vi "service_template.vi"() -> ()   [LabVIEW 2010]
panel:
  in  "password":string
  in  "username":string
  out "# elements in queue":i32
  out "error out":errorcluster
  in  "attributes":string[][](array[string])
  in  "Service Name":string
  in  "Network Manager IP Address or Hostname":string
  in  "timeout ms":i32=10000
  in  "Network Manager port":u16=1875
  # "NOTE: The function names and correspondng sub-VIs must be added to the case sequence on the block diagram."
  # "function name"
  # "function signature"
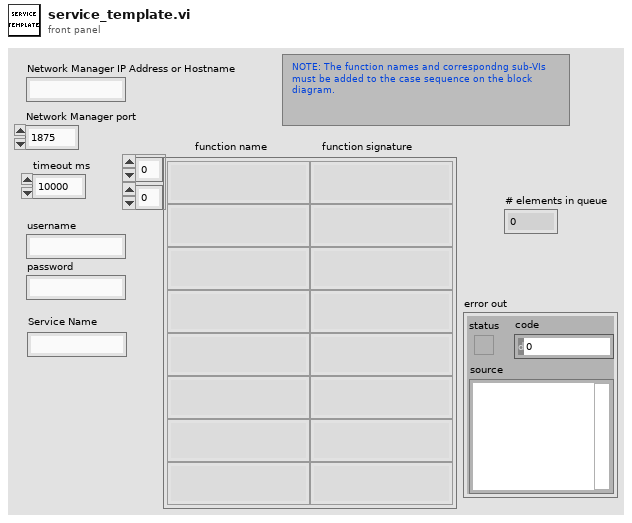
[diagram p1: front panel]
types:
  T1 = cluster{"type":u16, "name":string, "attributes":string[][]}
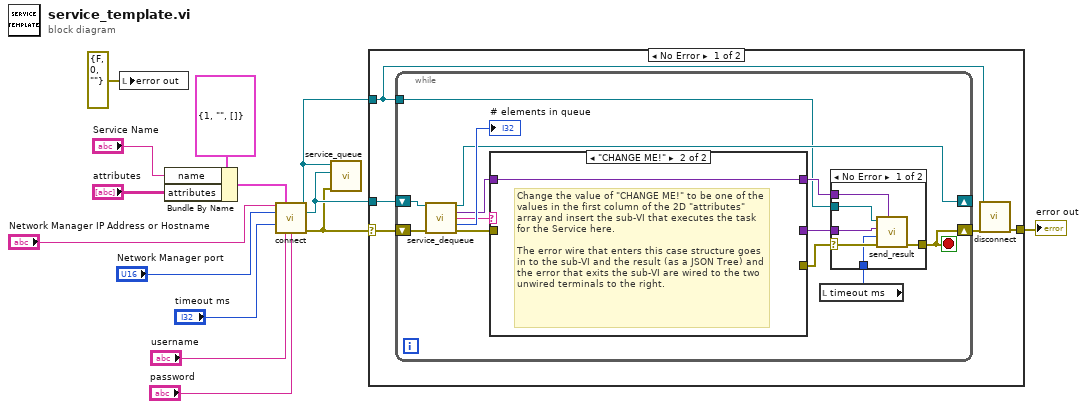
[diagram p0: block diagram]
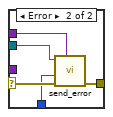
[diagram p2: hidden frame]
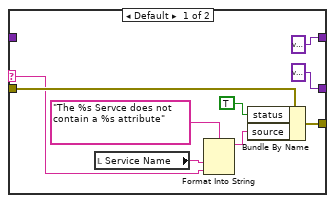
[diagram p3: hidden frame]
diagram:
  n1 = local write "error out"(errorcluster {"status"=FALSE, "code"=0, "source"=""} ("error out")) -> ()
  n2 = Bundle By Name(cluster=T1 {"type"=1, "name"="", "attributes"=[]} ("Identity"), "name"="Service Name", "attributes"="attributes") -> (w9:T1)
  n3 = call "connect.vi"("Network Manager IP Address or Hostname"="Network Manager IP Address or Hostname", "Identity"=w9, "Network Manager port"="Network Manager port", "timeout ms"="timeout ms", "username"="username", "password"="password") -> ("connection ID"=w5:refnum<k5>, "queue out"=w6:refnum<queue>, "error out"=w4:errorcluster)  [unwired: 7 in]
  n4 = call "service_queue.vi"("error in"=w4, "queue in"=w6, "connection ID"=w5) -> ()  [unwired: 9 in]
  n5 = case shown="No Error" w4 {
    selector: w4 -> [w15 w54]
    tunnel: w6 -> [w19 _]
    tunnel: w5 -> [w18 _]
    tunnel: [w16 w54] -> w3
    frame No Error {
      n6 = while {
        shift-right: [w31] -> w17
        shift-left: w15 -> [w29]
        shift-right: [w25] -> _
        shift-left: w19 -> [w30]
        tunnel: w18 -> [w20]
        stop <- w31 stop-if-true
        n7 = call "service_dequeue.vi"("queue"=w30, "error in"=w29) -> ("queue out"=w25:refnum<queue>, "JSON Tree Out Passthrough"=w24:variant, "function name"=w26:string, "# elements in queue"=→"# elements in queue":i32, "error out"=w28:errorcluster)  [unwired: 9 in]
        n8 = case shown="\"CHANGE ME!\"" w26 {
          selector: w26 -> [w47 _]
          tunnel: w28 -> [w52 _]
          tunnel: [w50 _] -> w32
          tunnel: w24 -> [_ w53]
          tunnel: [variant ("JSON Tree Out Passthrough") w53] -> w23
          tunnel: [variant ("result") _] -> w22
          frame Default {
            n9 = local read "Service Name"() -> (w48:string)
            n10 = Format Into String(format string="The %s Servce does not contain a %s attribute", w48, w47) -> (resulting string=w46:string)  [unwired: 2 in, 1 out]
            n11 = Bundle By Name(cluster=w52, "status"=TRUE, "source"=w46) -> (w50:errorcluster)
          }
          frame "CHANGE ME!" {
            # "Change the value of \"CHANGE ME!\" to be one of the values in the first column of the 2D \"attributes\" array and insert the sub-VI that executes the task for the Service here.\n\nThe error wire that enters this case structure goes in to the sub-VI and the result (as a JSON Tree) and the error that exits the sub-VI are wired to the two unwired terminals to the right."
          }
        }
        n12 = local read "timeout ms"() -> (w21:i32)
        n13 = case shown="No Error" w32 {
          selector: w32 -> [w38 w43]
          tunnel: [w37 w42] -> w31
          tunnel: w20 -> [w36 w41]
          tunnel: w23 -> [w35 w39]
          tunnel: w22 -> [w34 _]
          tunnel: w21 -> [w33 w40]
          frame No Error {
            n14 = call "send_result.vi"("JSON Tree In (JSON Object)"=w35, "error in"=w38, "timeout ms"=w33, "result"=w34, "connection ID"=w36) -> ("error out"=w37:errorcluster)  [unwired: 3 in, 3 out]
          }
          frame Error {
            n15 = call "send_error.vi"("JSON Tree In (JSON Object)"=w39, "error in"=w43, "timeout ms"=w40, "connection ID"=w41) -> ("error out"=w42:errorcluster)  [unwired: 4 in, 3 out]
          }
        }
      }
      n16 = call "disconnect.vi"("error in (no error)"=w17, "connection ID"=w18) -> ("error out"=w16:errorcluster)  [unwired: 9 in]
    }
    frame Error {
    }
  }
  "error out" <- w3
